vi "Get SMO PGSQL Log Paths.vi"(5 "getAll Cluster":variant, 7 "Default Paths":string, 8 "error in (no error)":errorcluster, 11 "Instrument.VRM in":refnum<class "Instrument.OxfordVRM.lvclass">) -> (0 "error out":errorcluster, 2 "Paths":string, 3 "Instrument.VRM out":refnum<class "Instrument.OxfordVRM.lvclass">)   [LabVIEW 2019, in "Instrument.OxfordVRM.lvclass"]
uses:
  Instrument.OxfordVRM.lvclass
  Typedefs/getAll.ctl
  <userlib>/LevyLab/Instrument Framework/Instrument Types/Cryostat/Instrument.Cryostat.lvclass
  <userlib>/LevyLab/LV-Data/LV-Data.PG/LV-Data.PGSQL.lvclass
  <userlib>/LevyLab/LV-Data/LV-Data.PG/API/Write Variable (one-row).vi
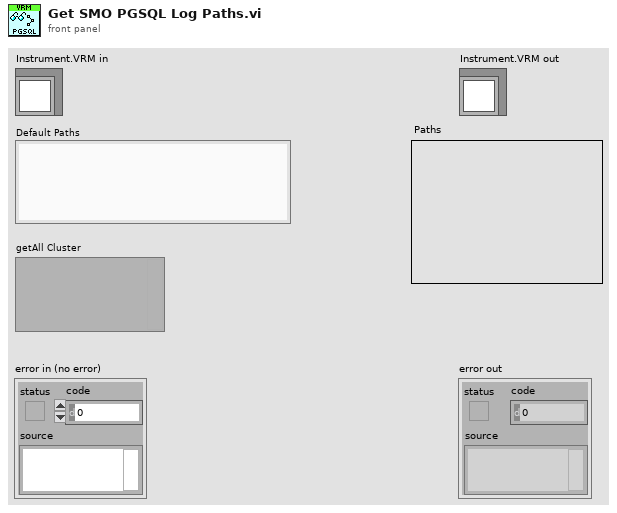
[diagram p1: front panel]
types:
  T1 = typedef "Instrument.OxfordVRM.lvclass/getAll.ctl" = cluster{"Field":dbl[], "Target Field":dbl[], "Target Field Rate":dbl[], "PSU Current":dbl[], "PSU Voltage":dbl[], "Status":string[]}
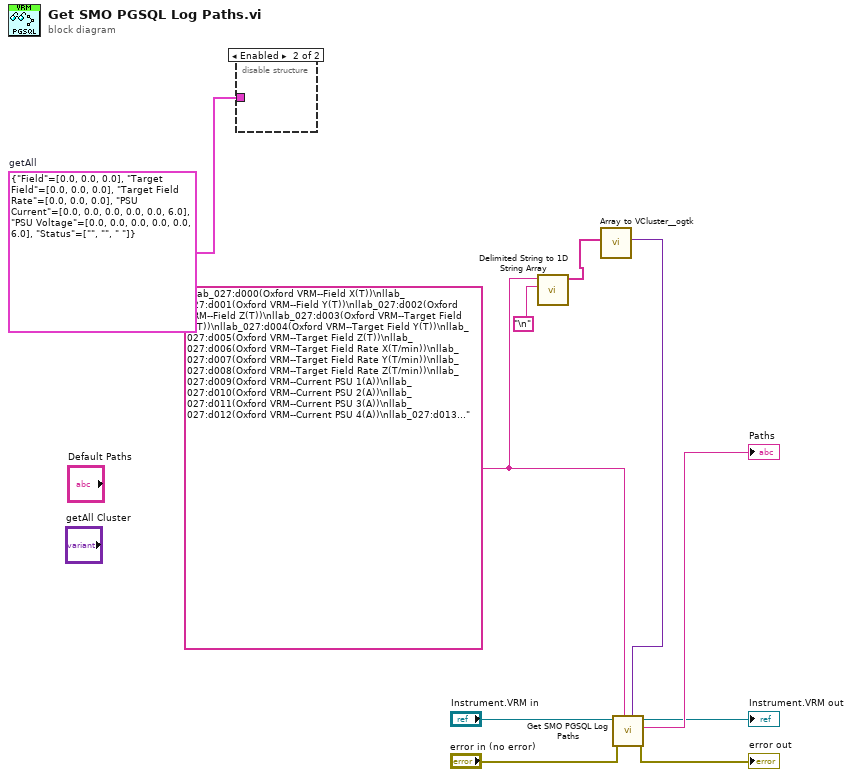
[diagram p0: block diagram]
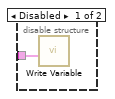
[diagram p2: hidden frame]
diagram:
  w4 = "llab_027:d000(Oxford VRM--Field X(T))\nllab_027:d001(Oxford VRM--Field Y(T))\nllab_027:d002(Oxford VRM--Field Z(T))\nllab_027:d003(Oxford VRM--Target Field X(T))\nllab_027:d004(Oxford VRM--Target Field Y(T))\nllab_027:d005(Oxford VRM--Target Field Z(T))\nllab_027:d006(Oxford VRM--Target Field Rate X(T/min))\nllab_027:d007(Oxford VRM--Target Field Rate Y(T/min))\nllab_027:d008(Oxford VRM--Target Field Rate Z(T/min))\nllab_027:d009(Oxford VRM--Current PSU 1(A))\nllab_027:d010(Oxford VRM--Current PSU 2(A))\nllab_027:d011(Oxford VRM--Current PSU 3(A))\nllab_027:d012(Oxford VRM--Current PSU 4(A))\nllab_027:d013(Oxford VRM--Current PSU 5(A))\nllab_027:d014(Oxford VRM--Current PSU 6(A))\nllab_027:d015(Oxford VRM--Voltage PSU 1(V))\nllab_027:d016(Oxford VRM--Voltage PSU 2(V))\nllab_027:d017(Oxford VRM--Voltage PSU 3(V))\nllab_027:d018(Oxford VRM--Voltage PSU 4(V))\nllab_027:d019(Oxford VRM--Voltage PSU 5(V))\nllab_027:d020(Oxford VRM--Voltage PSU 6(V))\nllab_027:v000(Oxford VRM--Status X())\nllab_027:v001(Oxford VRM--Status Y())\nllab_027:v002(Oxford VRM--Status Z())" ("Paths")
  w9 = T1 {"Field"=[0.0, 0.0, 0.0], "Target Field"=[0.0, 0.0, 0.0], "Target Field Rate"=[0.0, 0.0, 0.0], "PSU Current"=[0.0, 0.0, 0.0, 0.0, 0.0, 6.0], "PSU Voltage"=[0.0, 0.0, 0.0, 0.0, 0.0, 6.0], "Status"=["", "", " "]}  # getAll
  n1 = disable-structure shown="Enabled" {
    disable-tunnel: w9 -> [w11 _]
    frame Disabled {
      n2 = call-poly <userlib>:"Write Variable.vi"("Data"=w11) -> ()  [unwired: 7 in, 4 out]
    }
    frame Enabled {
    }
  }
  n3 = call <vilib>:"Delimited String to 1D String Array.vi"("delimiter"="\n", "delimited string"=w4) -> ("string array"=w2:string[])  [unwired: 9 in]
  n4 = call <userlib>:"Array to VCluster__ogtk.vi"("Array"=w2) -> ("VCluster"=w1:variant)  [unwired: 9 in, 1 out]
  n5 = call-parent "Get SMO PGSQL Log Paths.vi"("getAll Cluster"=w1, "Default Paths"=w4, "error in (no error)"="error in (no error)", "Instrument in"="Instrument.VRM in") -> ("error out"=→"error out":errorcluster, "Paths"=→"Paths":string, "Instrument out"=→"Instrument.VRM out":refnum<class "Instrument.OxfordVRM.lvclass">)  [unwired: 5 in]
